vi "ISO8601FileName.vi"(7 "Extension":string, 8 "error in (no error)":errorcluster, 9 "useUTC":bool, 10 "Timestamp":timestamp, 11 "BaseName":string) -> (0 "error out":errorcluster, 3 "FileName":string)   [LabVIEW 2026, in "Lumberjack.lvlib"]
doc: "Pure filename builder. Compose a log file name as an optional BaseName, an ISO\n8601 timestamp, and the extension, e.g. Pump_2026-07-06T143005.csv, or 2026-07-06T143005.csv when BaseName is empty (SRS-LMBR-035). UseUTC selects the frame (UTC vs local); colons in the time are removed for Windows and the text sorts lexically in chronological order. Extension is normalized: a leading dot is optional, so \"csv\" and \".csv\" both yield one dot, and an empty extension yields no trailing dot. Trusts inputs are valid (baseName is checked in Validate). Deterministic given inputs; no I/O."
uses:
  Lumberjack.lvlib
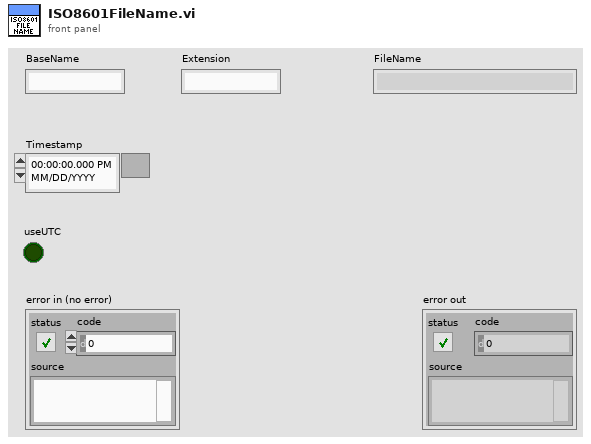
[diagram p1: front panel]
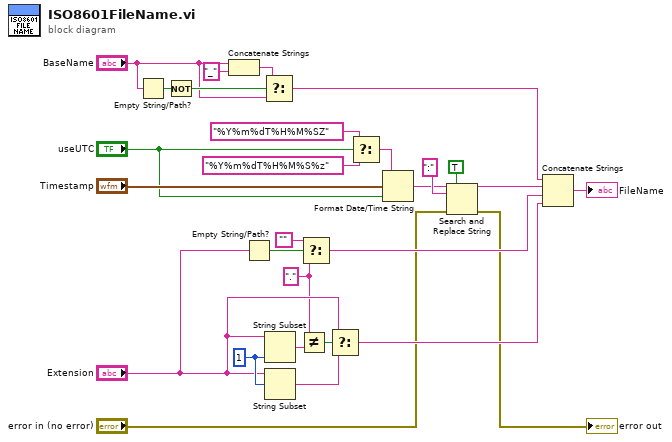
[diagram p0: block diagram]
diagram:
  w18 = 1 ("length (rest)")
  w10 = "." ("string")
  n1 = Empty String/Path?(string/path="BaseName") -> (empty?=w26:bool)
  n2 = Not(x=w26) -> (.not. x?=w25:bool)
  n3 = Concatenate Strings("BaseName", "_" ("string")) -> (w24:string)
  n4 = Empty String/Path?(string/path="Extension") -> (empty?=w11:bool)
  n5 = Select(t=w24, s=w25, f="BaseName") -> (s? t:f=w22:string)
  n6 = String Subset(string="Extension", length (rest)=w18) -> (substring=w21:string)  [unwired: 1 in]
  n7 = String Subset(string="Extension", offset (0)=w18) -> (substring=w17:string)  [unwired: 1 in]
  n8 = Not Equal?(x=w10, y=w21) -> (x != y?=w20:bool)
  n9 = Select(t="", s=w11, f=w10) -> (s? t:f=w9:string)
  n10 = Select(t="Extension", s=w20, f=w17) -> (s? t:f=w19:string)
  n11 = Select(t="%Y%m%dT%H%M%SZ" ("time format string (%c)"), s="useUTC", f="%Y%m%dT%H%M%S%z" ("time format string (%c)")) -> (s? t:f=w7:string)
  n12 = Format Date/Time String(time format string (%c)=w7, seconds (now)="Timestamp", UTC format="useUTC") -> (date/time string=w5:string)
  n13 = Search and Replace String(replace all?=TRUE ("replace all? (F)"), input string=w5, search string=":", error in="error in (no error)") -> (result string=w4:string, error out=→"error out":errorcluster)  [unwired: 4 in, 2 out]
  n14 = Concatenate Strings(w22, w4, w9, w19) -> (→"FileName":string)
